vi "setDefaultKickForce.vi"(8 "error in (no error)":errorcluster, 9 "KickForceMean":dbl[][](array[numeric]), 10 "InitialKickForce2DArray":dbl[][](array[numeric]), 11 "Game in":refnum<class "Game.lvclass">) -> (0 "error out":errorcluster, 2 "KickForceMeanWithDefaultKickForce":dbl[][](array[numeric]), 3 "Game out":refnum<class "Game.lvclass">)   [LabVIEW 2020, in "Game.lvclass"]
uses:
  Game.lvclass
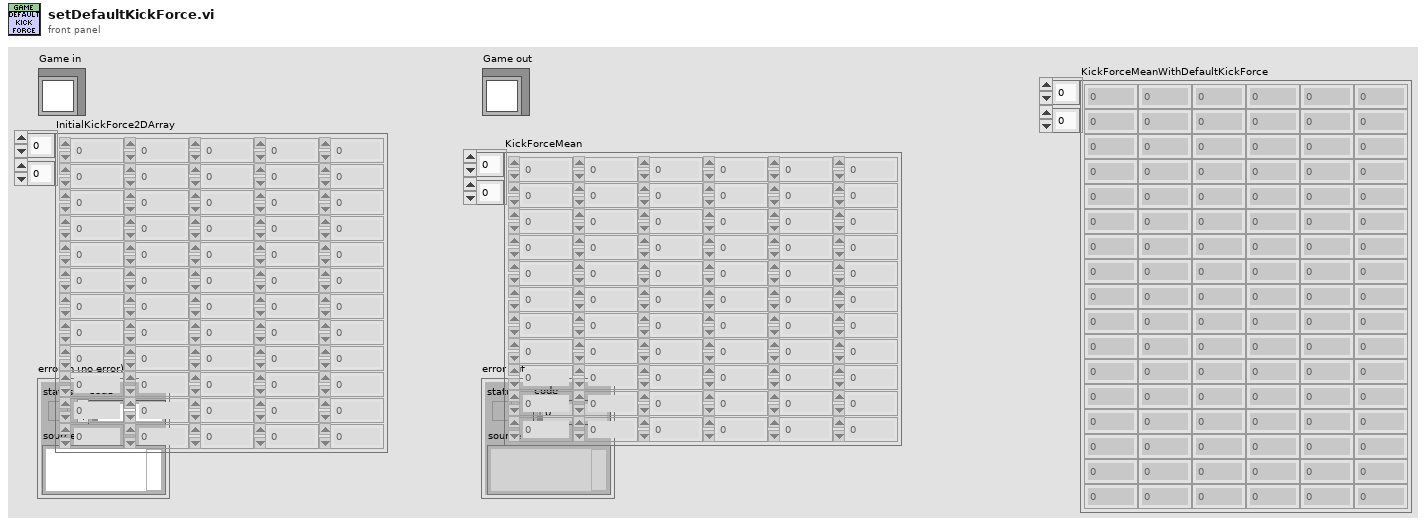
[diagram p1: front panel]
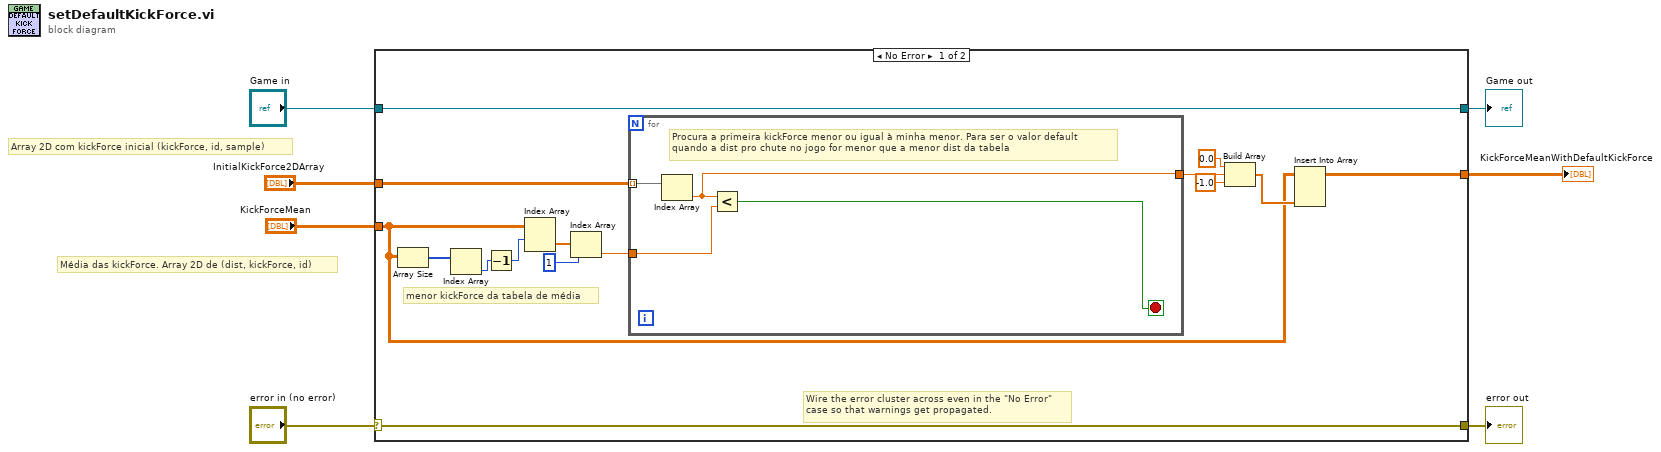
[diagram p0: block diagram]
diagram:
  # "Média das kickForce. Array 2D de (dist, kickForce, id)"
  # "Array 2D com kickForce inicial (kickForce, id, sample)"
  n1 = case shown="No Error" "error in (no error)" {
    selector: "error in (no error)" -> [w21 w28]
    tunnel: [w21 w28] -> w6
    tunnel: [w22 w27] -> w4
    tunnel: "Game in" -> [w22 w27]
    tunnel: "InitialKickForce2DArray" -> [w20 _]
    tunnel: "KickForceMean" -> [w11 _]
    tunnel: [w10 _] -> w1
    frame No Error {
      # "menor kickForce da tabela de média"
      # "Wire the error cluster across even in the \"No Error\"\ncase so that warnings get propagated."
      n2 = Array Size(array=w11) -> (size(s)=w19:i32[])
      n3 = Index Array(array=w19) -> (element=w9:i32)  [unwired: 1 in]
      n4 = Decrement(x=w9) -> (x-1=w8:i32)
      n5 = Index Array(array=w11, index (row)=w8) -> (element=w18:dbl[])  [unwired: 1 in]
      n6 = Index Array(array=w18, index=1) -> (element=w16:dbl)
      n7 = for {
        tunnel: w20 -> [w26] mode=indexing
        tunnel: w16 -> [w25]
        tunnel: [w23] -> w14
        stop <- w24 stop-if-true
        # "Procura a primeira kickForce menor ou igual à minha menor. Para ser o valor default\nquando a dist pro chute no jogo for menor que a menor dist da tabela"
        n8 = Index Array(array=w26) -> (element=w23:dbl)  [unwired: 1 in]
        n9 = Less?(x=w23, y=w25) -> (x < y?=w24:bool)
      }
      n10 = Build Array(0.0 ("element"), w14, -1.0 ("element")) -> (w12:dbl[])
      n11 = Insert Into Array(array=w11, new element=w12) -> (w10:dbl[][])  [unwired: 2 in]
    }
    frame Error {
    }
  }
  "error out" <- w6
  "Game out" <- w4
  "KickForceMeanWithDefaultKickForce" <- w1
